vi "CCE RRMA P03 SubVI09.vi"(11 "MOMENTOS INVARIANTES DE HU":dbl[](array[numeric])=[0.9997525383124077, 0.022047103684425993, 0.00047771658598479535, 0.0029255984598577215, 8.143259107920102e-07, 4.0976510303173995e-06, -2.948715981189433e-07]) -> (0 "logical OR":bool, 1 "Array":dbl[](array[numeric]), 2 "min value":dbl, 3 "element":string)   [LabVIEW 2020]
doc: "Ceballos Conde Emanuel Rodríguez Ramírez Miguel Ángel 4MV6 Sistemas de visión artificial 2022/1\nEste vi contiene el funcionamiento de una neurona compet y a su vez la memoria que esta requiere para operar, este vi da como resultado el nombre del objeto en memoria que detecte la neurona respecto a la entrada"
panel:
  out "appended array":dbl[][](array[numeric])
  # "Ceballos Conde Emanuel\nRodríguez Ramírez Miguel Ángel\n4MV6\nSistemas de visión artificial\n2022/1"
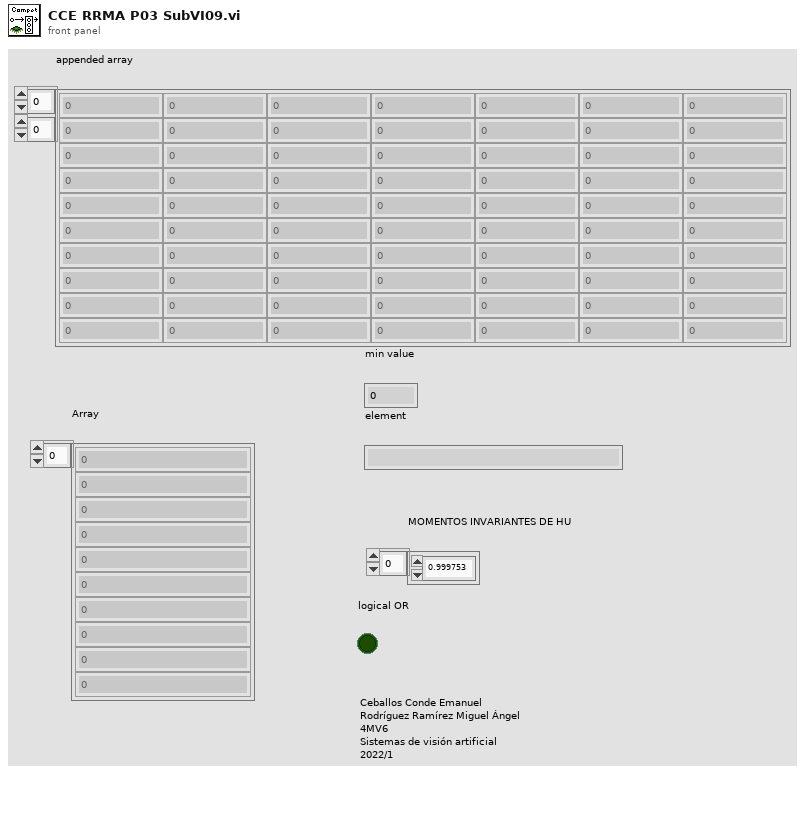
[diagram p1: front panel]
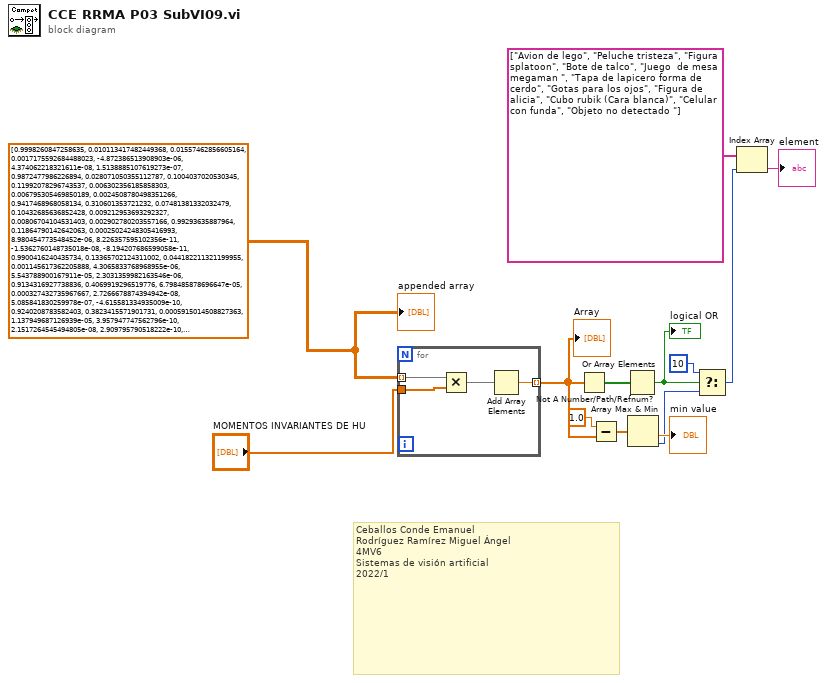
[diagram p0: block diagram]
diagram:
  w1 = dbl[][] [[0.9998260847258635, 0.010113417482449368, 0.01557462856605164, 0.0017175592684488023, -4.872386513908903e-06, 4.374062218321611e-08, 1.5138885107619273e-07], [0.9872477986226894, 0.028071050355112787, 0.1004037020530345, 0.11992078296743537, 0.006302356185858303, 0.006795305469850189, 0.0024508780498351266], [0.9417468968058134, 0.310601353721232, 0.07481381332032479, 0.10432685636852428, 0.009212953693292327, 0.00806704104531403, 0.002902780203557166], [0.99293635887964, 0.11864790142642063, 0.00025024248305416993, 8.980454773548452e-06, 8.226357595102356e-11, -1.5362760148735018e-08, -8.194207686599058e-11], [0.9900416240435734, 0.13365702124311002, 0.044182211321199955, 0.001145617362205888, 4.3065833768968955e-06, 5.543788900167911e-05, 2.3031359982163546e-06], [0.9134316927738836, 0.4069919296519776, 6.798485878696647e-05, 0.000327432735967667, 2.7266678874394942e-08, 5.085841830259978e-07, -4.615581334935009e-10], [0.9240208783582403, 0.3823415571901731, 0.0005915014508827363, 1.137949687126939e-05, 3.957947747562796e-10, 2.1517264545494805e-08, 2.909795790518222e-10], [0.994765613853628, 0.09732221757456085, 0.03041456649378277, 0.006686772050812854, 2.6007594020255687e-05, 2.429188291092389e-06, -1.7390671348546814e-06], [0.9999997080867683, 0.0007640583488216332, 4.551103422565089e-06, 4.52827510295342e-06, -2.6965238360993628e-12, 4.7224332350655394e-09, 3.3275233672116626e-12], [0.9966873842602609, 0.08132807302127802, 4.16091732179383e-05, 2.9389523630263203e-05, 2.085257405688756e-10, -1.3144628336867574e-07, -9.814620585741512e-11]] ("MOMENTOS INVARIANTES DE HU")
  # "Ceballos Conde Emanuel\nRodríguez Ramírez Miguel Ángel\n4MV6\nSistemas de visión artificial\n2022/1"
  n1 = for {
    tunnel: w1 -> [w17] mode=indexing
    tunnel: "MOMENTOS INVARIANTES DE HU" -> [w16]
    tunnel: [w14] -> w7 mode=indexing
    n2 = Multiply(x=w17, y=w16) -> (x*y=w15:dbl[])
    n3 = Add Array Elements(numeric array=w15) -> (sum=w14:dbl)
  }
  "Array" <- w7
  n4 = Not A Number/Path/Refnum?(number/path/refnum=w7) -> (NaN/Path/Refnum?=w5:bool[])
  n5 = Subtract(x=1.0, y=w7) -> (x-y=w12:dbl[])
  n6 = Or Array Elements(Boolean array=w5) -> (logical OR=w6:bool)
  "logical OR" <- w6
  n7 = Array Max & Min(array=w12) -> (min value=→"min value":dbl, min index (indices)=w3:i32)  [unwired: 2 out]
  n8 = Select(t=10, s=w6, f=w3) -> (s? t:f=w4:i32)
  n9 = Index Array(array=string[] ["Avion de lego", "Peluche tristeza", "Figura splatoon", "Bote de talco", "Juego  de mesa megaman ", "Tapa de lapicero forma de cerdo", "Gotas para los ojos", "Figura de alicia", "Cubo rubik (Cara blanca)", "Celular con funda", "Objeto no detectado "], index=w4) -> (element=→"element":string)
  "appended array" <- w1
